vi "ep_Power Correction (IEC).vi"(8 "error in (no error)":errorcluster, 9 "voltage MN values":dbl[](array[numeric]), 10 "voltage RMS values":dbl[](array[numeric]), 11 "power values":T1[](array[typedef])) -> (0 "error out":errorcluster, 2 "calibrated active power":dbl[](array[numeric]), 3 "dup power values":T1[](array[typedef]))   [LabVIEW 2024]
doc: "Calibrate the active power according to IEC76-1(1993)."
uses:
  <vilib>/addons/Electrical Power/Basic/Measurement/subVIs/basic_Power Value.ctl
  <vilib>/addons/Electrical Power/Basic/NI_EP_Basic.lvlib
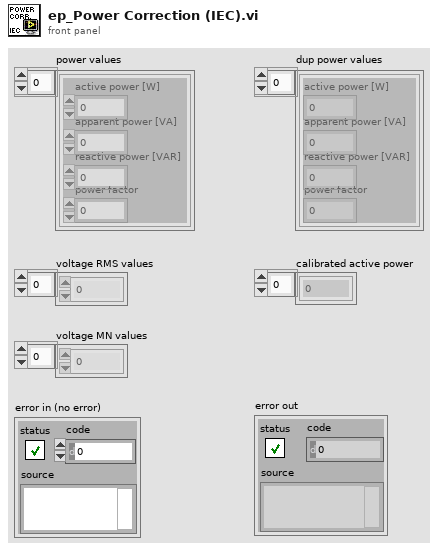
[diagram p1: front panel]
types:
  T1 = typedef "NI_EP_Basic.lvlib/basic_Power Value.ctl" = cluster{"active power [W]":dbl, "apparent power [VA]":dbl, "reactive power [VAR]":dbl, "power factor":dbl}
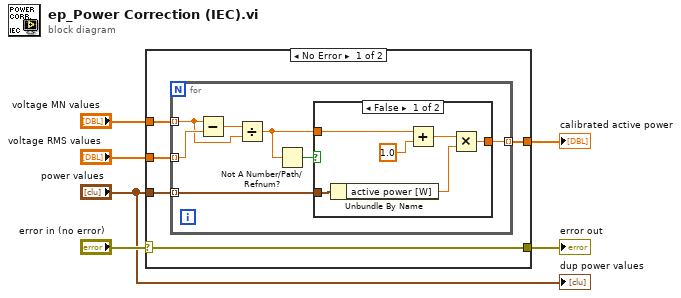
[diagram p0: block diagram]
diagram:
  n1 = case shown="No Error" "error in (no error)" {
    selector: "error in (no error)" -> [w7 w25]
    tunnel: "power values" -> [w11 _]
    tunnel: "voltage MN values" -> [w10 _]
    tunnel: "voltage RMS values" -> [w9 _]
    tunnel: [w8 _] -> w3
    tunnel: [w7 w25] -> w2
    frame No Error {
      n2 = for {
        tunnel: w11 -> [w18] mode=indexing
        tunnel: w10 -> [w15] mode=indexing
        tunnel: w9 -> [w17] mode=indexing
        tunnel: [w14] -> w8 mode=indexing
        n3 = Subtract(x=w15, y=w17) -> (x-y=w16:dbl)
        n4 = Divide(x=w16, y=w15) -> (x/y=w12:dbl)
        n5 = Not A Number/Path/Refnum?(number/path/refnum=w12) -> (NaN/Path/Refnum?=w13:bool)
        n6 = case shown="False" w13 {
          tunnel: w18 -> [w24 _]
          tunnel: w12 -> [w23 _]
          tunnel: [w19 _] -> w14
          frame False {
            n7 = Unbundle By Name(w24) -> ("active power [W]"=w20:dbl)
            n8 = Add(x=w23, y=1.0) -> (x+y=w21:dbl)
            n9 = Multiply(x=w21, y=w20) -> (x*y=w19:dbl)
          }
          frame True {
          }
        }
      }
    }
    frame Error {
    }
  }
  "error out" <- w2
  "calibrated active power" <- w3
  "dup power values" <- "power values"
